vi "Geometry.vi"(11 "DeviceType":string) -> (3 "MFG":i32)   [LabVIEW 2015]
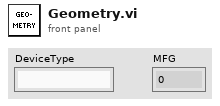
[diagram p1: front panel]
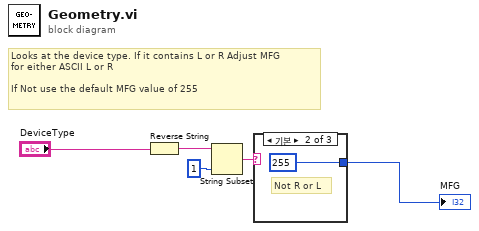
[diagram p0: block diagram]
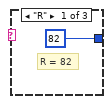
[diagram p2: hidden frame]
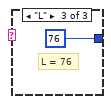
[diagram p3: hidden frame]
diagram:
  # "Looks at the device type. If it contains L or R Adjust MFG\nfor either ASCII L or R\n\nIf Not use the default MFG value of 255"
  n1 = Reverse String(1:"DeviceType") -> (0:w4:string)
  n2 = String Subset(string=w4, length (rest)=1) -> (substring=w3:string)  [unwired: 1 in]
  n3 = case shown="기본" w3 {
    tunnel: [82 255 76] -> w1
    frame "R" {
      # "R = 82"
    }
    frame Default {
      # "Not R or L"
    }
    frame "L" {
      # "L = 76"
    }
  }
  "MFG" <- w1
